vi "Read Unified Msg Set.vi"(11 "Base Attributes in":refnum<class "Base Attributes.lvclass">) -> (2 "Unified Msg Set":T1)   [LabVIEW 2025, in "jettl.lvlib" / "Base Attributes.lvlib" / "Base Attributes.lvclass"]
uses:
  Base Attributes.lvclass
  Msg Set.ctl
  Msg/Msg.lvclass
  Base Attributes.lvclass/Base Attributes.ctl
  jettl.lvlib
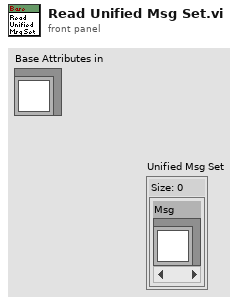
[diagram p1: front panel]
types:
  T1 = typedef "jettl.lvlib/Msg Set.ctl" = set{refnum<class "Msg.lvclass">}
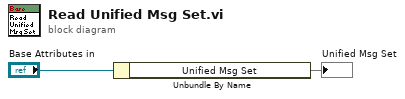
[diagram p0: block diagram]
diagram:
  n1 = Unbundle By Name("Base Attributes in") -> ("Unified Msg Set"=→"Unified Msg Set":T1)
